vi "Current Probe.vi"(0 "object in":refnum<class "TBS2000Series.lvclass">, 5 "error in (no error)":errorcluster) -> (14 "object out":refnum<class "TBS2000Series.lvclass">, 16 "Current Probe":T1(graph), 19 "error out":errorcluster)   [LabVIEW 2023, in "TBS2000Series.lvclass"]
uses:
  TBS2000Series.lvclass
  TBS2000Series.lvclass/TBS2000Series.ctl
  <instrlib>/Tektronix TBS 2000 Series/Tektronix TBS 2000 Series.lvlib
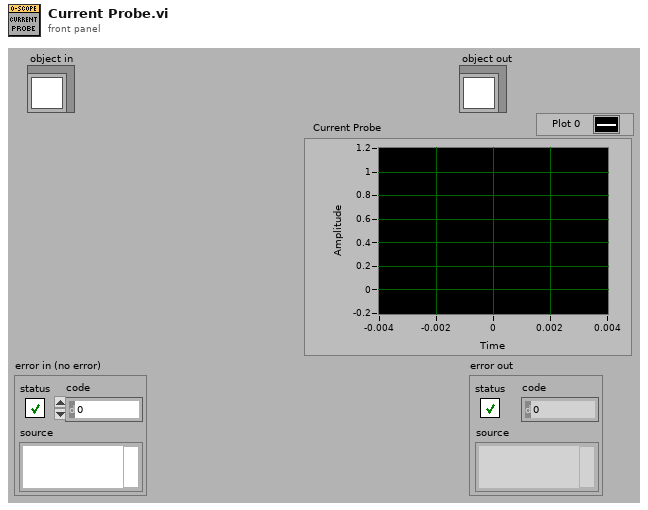
[diagram p1: front panel]
types:
  T1 = cluster{"Initial X":dbl, "X Increment":dbl, "Waveform Array":dbl[]}
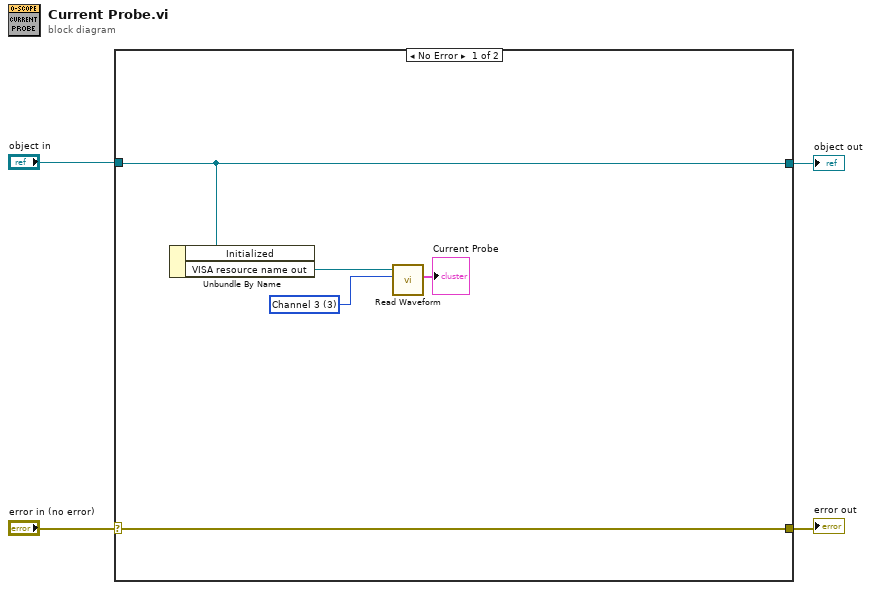
[diagram p0: block diagram]
diagram:
  n1 = case shown="No Error" "error in (no error)" {
    selector: "error in (no error)" -> [w9 w11]
    tunnel: [w9 w11] -> w3
    tunnel: [w6 w10] -> w1
    tunnel: "object in" -> [w6 w10]
    frame No Error {
      w7 = 3 items=["Math", "Channel 1", "Channel 2", "Channel 3", "Channel 4"] ("Source (1: Channel 1)")
      n2 = Unbundle By Name(w6) -> ("VISA resource name out"=w8:refnum<visa-resource-name>)  [unwired: 1 out]
      n3 = call <instrlib>:"Read Waveform.vi"("Source (1: Channel 1)"=w7, "VISA resource name"=w8) -> ("Waveform Graph"=→"Current Probe":T1)  [unwired: 7 in, 2 out]
    }
    frame Error {
    }
  }
  "error out" <- w3
  "object out" <- w1
